vi "UTF Time Measurement Runner.vi"() -> ()   [LabVIEW 2018]
uses:
  <vilib>/utf/common/utf_test_result.ctl
  Common Support/Test File Path--cluster.ctl
  Common Support/Common Support.lvlib
  <vilib>/utf/NI_UnitTestFramework.lvlib
panel:
  in  "Calculate Temperature Change":bool=TRUE
  in  "Thermal Chamber Response Simulator_Init":bool=TRUE
  in  "Get Chamber Status":bool=TRUE
  in  "GUI Interlock Tester":bool=TRUE
  in  "Convert Shutdown Furnace to Heater State Enum":bool=TRUE
  in  "Action Update Ramp Rate":bool=TRUE
  in  "Action Update Set Point":bool=TRUE
  in  "Action Update Heater State":bool=TRUE
  in  "All Test":bool
  out "UTF In Progress":bool
  out "UTF Testing time (seconds)":dbl
  out "UTF Results":T1[](array[typedef])
  in  "Multiplier of runs":i32=10
  out "No. of Tests":i32=10
  # "If \"All Test\" is true, then all of selected and unselected tests \nbelow will be executed and each test will be executed only \nonce independently of \"Multiplier of runs\"."
  # "UTF"
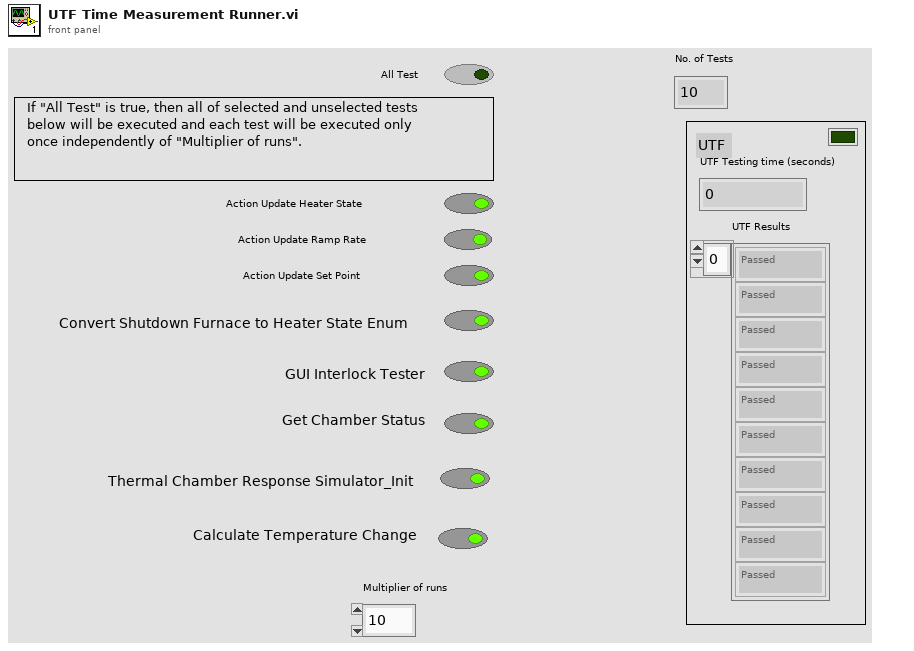
[diagram p1: front panel]
types:
  T1 = typedef "NI_UnitTestFramework.lvlib/utf_test_result.ctl" = enum16{"Passed", "Failed", "Error", "Skipped", "Not Processed"}
  T2 = typedef "Common Support.lvlib/Test File Path--cluster.ctl" = cluster{"Folder Name":string, "Test File Name":string}
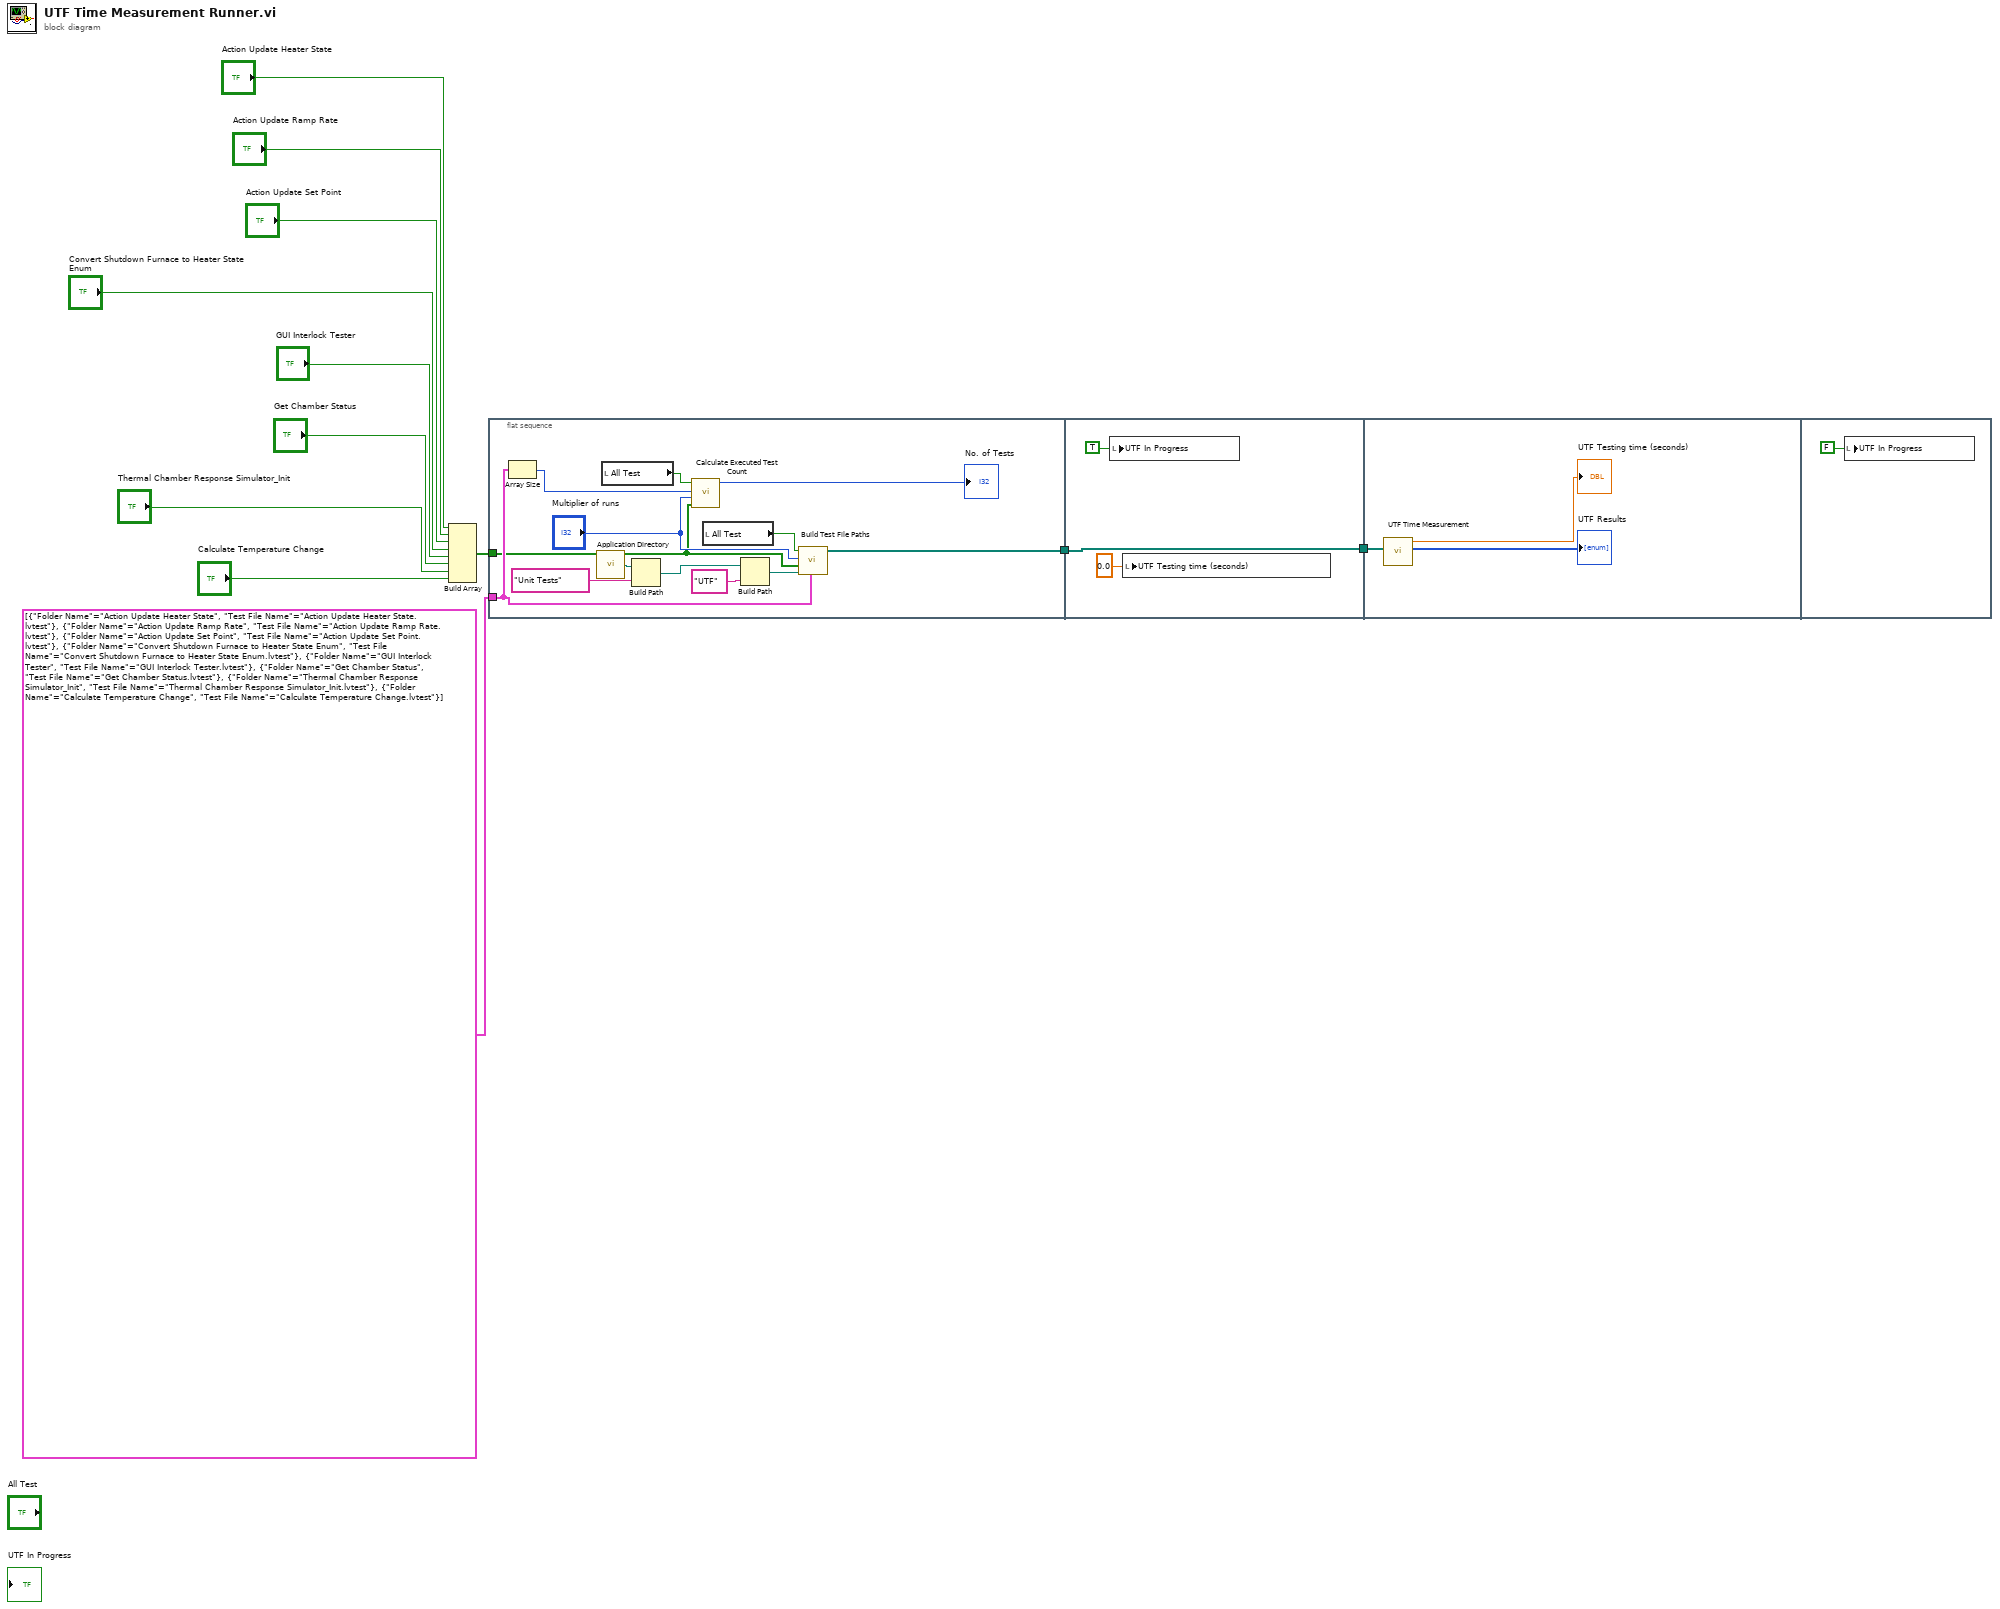
[diagram p0: block diagram]
diagram:
  n1 = Build Array("Action Update Heater State", "Action Update Ramp Rate", "Action Update Set Point", "Convert Shutdown Furnace to Heater State Enum", "GUI Interlock Tester", "Get Chamber Status", "Thermal Chamber Response Simulator_Init", "Calculate Temperature Change") -> (w4:bool[])
  n2 = flat-sequence {
    tunnel: T2[] [{"Folder Name"="Action Update Heater State", "Test File Name"="Action Update Heater State.lvtest"}, {"Folder Name"="Action Update Ramp Rate", "Test File Name"="Action Update Ramp Rate.lvtest"}, {"Folder Name"="Action Update Set Point", "Test File Name"="Action Update Set Point.lvtest"}, {"Folder Name"="Convert Shutdown Furnace to Heater State Enum", "Test File Name"="Convert Shutdown Furnace to Heater State Enum.lvtest"}, {"Folder Name"="GUI Interlock Tester", "Test File Name"="GUI Interlock Tester.lvtest"}, {"Folder Name"="Get Chamber Status", "Test File Name"="Get Chamber Status.lvtest"}, {"Folder Name"="Thermal Chamber Response Simulator_Init", "Test File Name"="Thermal Chamber Response Simulator_Init.lvtest"}, {"Folder Name"="Calculate Temperature Change", "Test File Name"="Calculate Temperature Change.lvtest"}] -> [w14]
    tunnel: [w19] -> w6
    tunnel: w4 -> [w13]
    tunnel: w6 -> [w26]
    tunnel: [w26] -> w5
    tunnel: w5 -> [w29]
    frame #0 {
      n3 = Array Size(array=w14) -> (size(s)=w15:i32)
      n4 = call <vilib>:"Application Directory.vi"() -> ("Application Directory"=w25:path)
      n5 = local read "All Test"() -> (w17:bool)
      n6 = Build Path(base path=w25, name or relative path="Unit Tests") -> (appended path=w22:path)
      n7 = call "Calculate Executed Test Count.vi"("Test Selector Array"=w13, "Multiplier of Runs"="Multiplier of runs", "All Test Count"=w15, "Run All Tests"=w17) -> ("Executed Test Count"=→"No. of Tests":i32)  [unwired: 7 in]
      n8 = local read "All Test"() -> (w21:bool)
      n9 = Build Path(base path=w22, name or relative path="UTF") -> (appended path=w20:path)
      n10 = call "Build Test File Paths.vi"("Test Files"=w14, "Tests Folder Path"=w20, "Runnable Test Selector"=w13, "Multiplier of runs"="Multiplier of runs", "Run All"=w21) -> ("Test File Paths to Execute"=w19:path[])  [unwired: 6 in]
    }
    frame #1 {
      n11 = local write "UTF In Progress"(TRUE) -> ()
      n12 = local write "UTF Testing time (seconds)"(0.0) -> ()
    }
    frame #2 {
      n13 = call "UTF Time Measurement.vi"("test file paths"=w29) -> ("UTF Results"=→"UTF Results":T1[], "UTF Testing time (seconds)"=→"UTF Testing time (seconds)":dbl)  [unwired: 9 in]
    }
    frame #3 {
      n14 = local write "UTF In Progress"(FALSE) -> ()
    }
  }
